vi "get_smith_hover.vi"(4 "smith_pos_left":i32, 5 "left_center":dbl, 6 "smith_pos_top":i32, 7 "top_center":dbl, 8 "Coords":T2, 10 "cursor_data":cluster{"array type (2D Dbl)":dbl[], dbl[]}[](array[cluster]), 11 "ref_data":cluster{"array type (2D Dbl)":dbl[], dbl[]}[](array[cluster])) -> (0 "cursor_pos":cluster{"r_norm":dbl, "x_norm":dbl}, 3 "cursor_data":T1)   [LabVIEW 2025]
uses:
  <vilib>/Utility/miscctls.llb/LVPoint32TypeDef.ctl
panel:
  out "curs_x":dbl format="%0.2f"
  out "curs_r":dbl format="%0.2f"
  out "phase":dbl
  out "frequency":dbl
  out "r":dbl
  out "jx":dbl
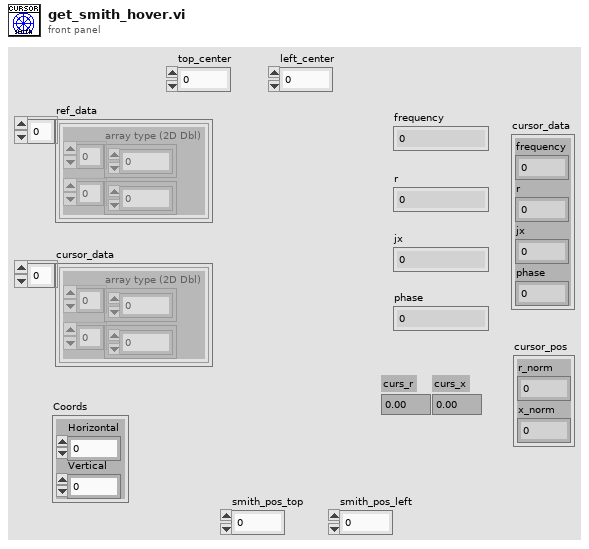
[diagram p1: front panel]
types:
  T1 = cluster{"frequency":dbl, "r":dbl, "jx":dbl, "phase":dbl}
  T2 = typedef "LVPoint32TypeDef.ctl" = cluster{"Horizontal":i32, "Vertical":i32}
  T3 = cluster{dbl, "phase":dbl, "phase":dbl, "phase":dbl}
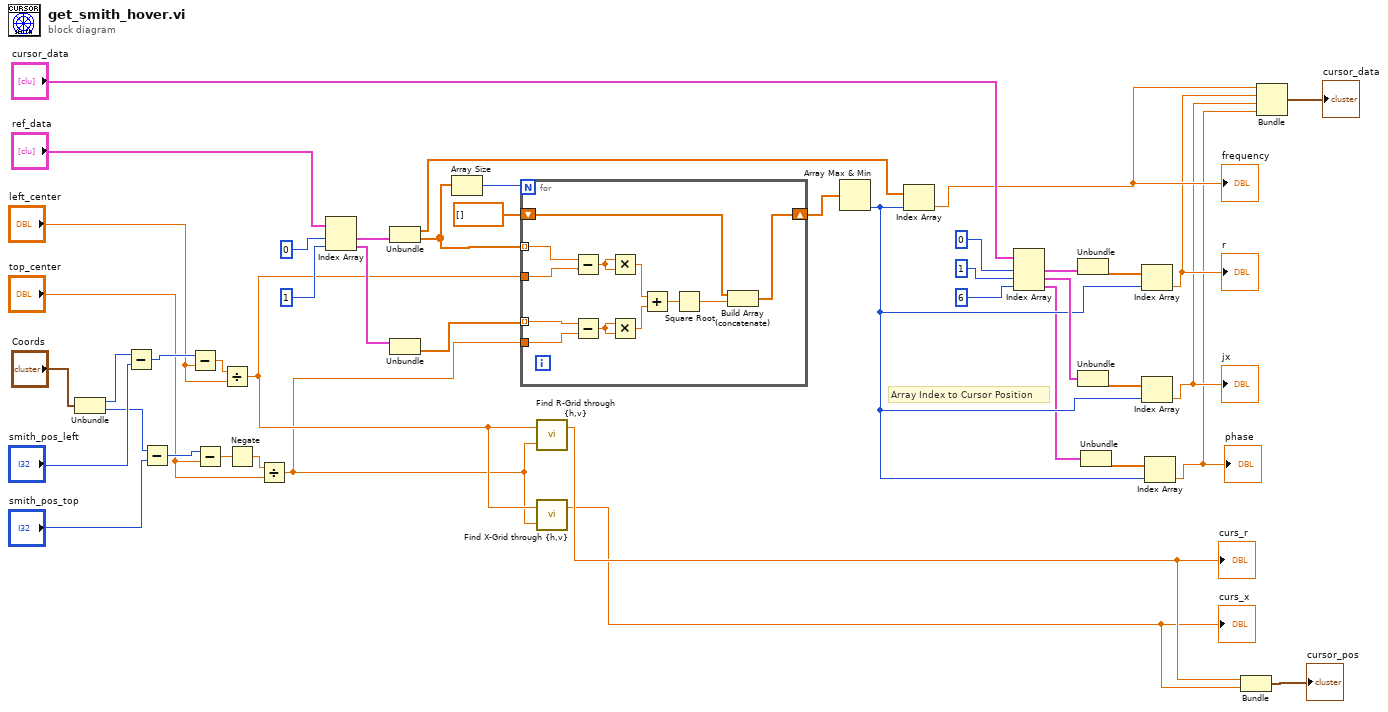
[diagram p0: block diagram]
diagram:
  # "Array Index to Cursor Position"
  n1 = Unbundle("Coords") -> ("Horizontal"=w28:i32, "Vertical"=w32:i32)
  n2 = Subtract(x=w28, y="smith_pos_left") -> (x-y=w29:i32)
  n3 = Subtract(x=w32, y="smith_pos_top") -> (x-y=w31:i32)
  n4 = Subtract(x=w29, y="left_center") -> (x-y=w30:dbl)
  n5 = Subtract(x=w31, y="top_center") -> (x-y=w33:dbl)
  n6 = Divide(x=w30, y="left_center") -> (x/y=w10:dbl)
  n7 = Negate(x=w33) -> (-x=w34:dbl)
  n8 = Divide(x=w34, y="top_center") -> (x/y=w9:dbl)
  n9 = Index Array(array="ref_data", index #1=0 ("index"), index #2=1 ("index")) -> (element #1=w14:cluster{"array type (2D Dbl)":dbl[], dbl[]}, element #2=w25:cluster{"array type (2D Dbl)":dbl[], dbl[]})
  n10 = Unbundle(w14) -> ("array type (2D Dbl)"=w13:dbl[], w11:dbl[])
  n11 = Unbundle(w25) -> (w12:dbl[])  [unwired: 1 out]
  n12 = Array Size(array=w11) -> (size(s)=w38:i32)
  n13 = for {
    N: w38 -> [_]
    tunnel: w11 -> [w54] mode=indexing
    tunnel: w12 -> [w56] mode=indexing
    tunnel: w9 -> [w55]
    tunnel: w10 -> [w53]
    shift-right: [w45] -> w40
    shift-left: dbl[] [] -> [w47]
    n14 = Subtract(x=w54, y=w53) -> (x-y=w52:dbl)
    n15 = Subtract(x=w56, y=w55) -> (x-y=w51:dbl)
    n16 = Multiply(x=w52, y=w52) -> (x*y=w49:dbl)
    n17 = Multiply(x=w51, y=w51) -> (x*y=w50:dbl)
    n18 = Add(x=w49, y=w50) -> (x+y=w48:dbl)
    n19 = Square Root(x=w48) -> (sqrt(x)=w46:dbl)
    n20 = Build Array (concatenate)(w47, w46) -> (w45:dbl[])
  }
  n21 = call <vilib>:"Find R-Grid through {h,v}.vi"("v"=w9, "h"=w10) -> ("R"=w3:dbl)  [unwired: 1 out]
  "curs_r" <- w3
  n22 = call <vilib>:"Find X-Grid through {h,v}.vi"("v"=w9, "h"=w10) -> ("x"=w2:dbl)  [unwired: 1 out]
  "curs_x" <- w2
  n23 = Array Max & Min(array=w40) -> (min index (indices)=w17:i32)  [unwired: 3 out]
  n24 = Index Array(array=w13, index=w17) -> (element=w8:dbl)
  "frequency" <- w8
  n25 = Index Array(array="cursor_data", index #1=0 ("index"), index #2=1 ("index"), index #3=6 ("index")) -> (element #1=w41:cluster{"array type (2D Dbl)":dbl[], dbl[]}, element #2=w23:cluster{"array type (2D Dbl)":dbl[], dbl[]}, element #3=w16:cluster{"array type (2D Dbl)":dbl[], dbl[]})
  n26 = Unbundle(w41) -> (w43:dbl[])  [unwired: 1 out]
  n27 = Unbundle(w23) -> (w44:dbl[])  [unwired: 1 out]
  n28 = Unbundle(w16) -> (w18:dbl[])  [unwired: 1 out]
  n29 = Index Array(array=w43, index=w17) -> (element=w7:dbl)
  "r" <- w7
  n30 = Index Array(array=w44, index=w17) -> (element=w6:dbl)
  "jx" <- w6
  n31 = Index Array(array=w18, index=w17) -> (element=w5:dbl)
  "phase" <- w5
  n32 = Bundle("R"=w3, "x"=w2) -> (→"cursor_pos":cluster{"R":dbl, "x":dbl})  [unwired: 1 in]
  n33 = Bundle(w8, "phase"=w7, "phase"=w6, "phase"=w5) -> (→"cursor_data":T3)  [unwired: 1 in]
